vi "Display Help Dialog.vi"(8 "error in (no error)":errorcluster, 10 "Help Text":string, 11 "CCD Configuration in":refnum<class "CCD Configuration.lvclass">) -> (0 "error out":errorcluster, 3 "CCD Configuration out":refnum<class "CCD Configuration.lvclass">)   [LabVIEW 2016, in "Hardware.lvlib" / "CCD.lvlib" / "CCD Configuration.lvclass"]
uses:
  <userlib>/Common Components/Hardware/CCD/CCD Configuration.lvclass
  <userlib>/Configuration Dialog Actor/Configuration.lvclass
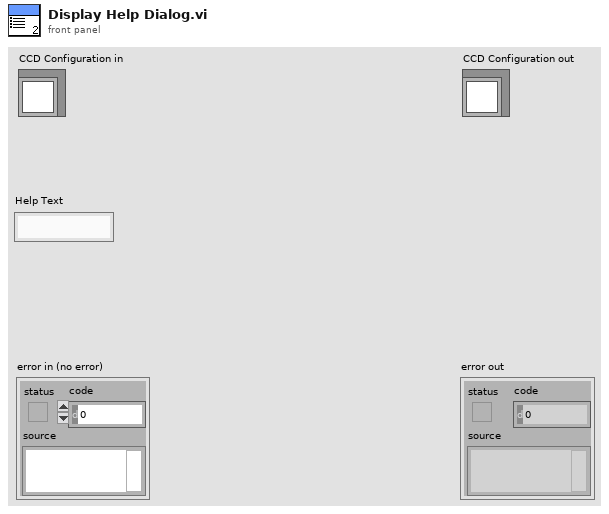
[diagram p1: front panel]
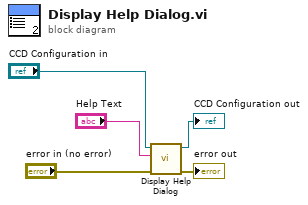
[diagram p0: block diagram]
diagram:
  n1 = call-parent "Display Help Dialog.vi"("error in (no error)"="error in (no error)", "Help Text"="Help Text", "Configuration in"="CCD Configuration in") -> ("error out"=→"error out":errorcluster, "Configuration out"=→"CCD Configuration out":refnum<class "CCD Configuration.lvclass">)  [unwired: 7 in]
